vi "Read Data.vi"(8 "error in (no error)":errorcluster, 11 "DLP2 in":refnum<class "DLP2.lvclass">) -> (0 "error out":errorcluster, 2 "DLP2ReadData":T1, 3 "DLP2 out":refnum<class "DLP2.lvclass">)   [LabVIEW 2022 SP3, in "DLP2.lvclass"]
doc: "Developed by Kevin Thompson\nkevin@thompsonengineering.net\n\nCopyright 2018\nThompson Engineering, LLC"
uses:
  DLP2.lvclass
  DataTypes/Read Data--cluster.ctl
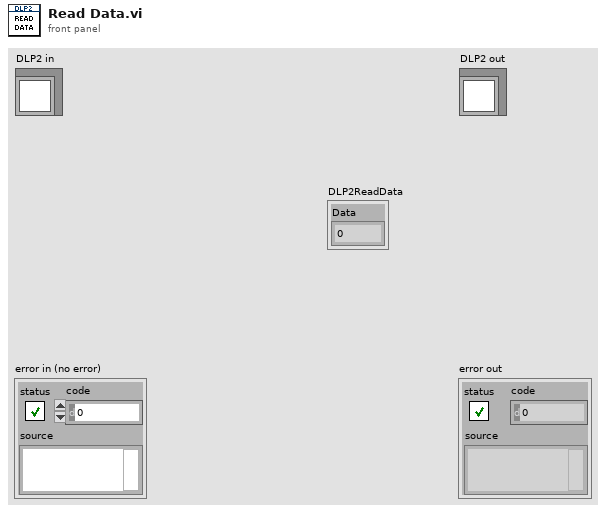
[diagram p1: front panel]
types:
  T1 = typedef "DLP2.lvclass/Read Data--cluster.ctl" = cluster{"Data":dbl}
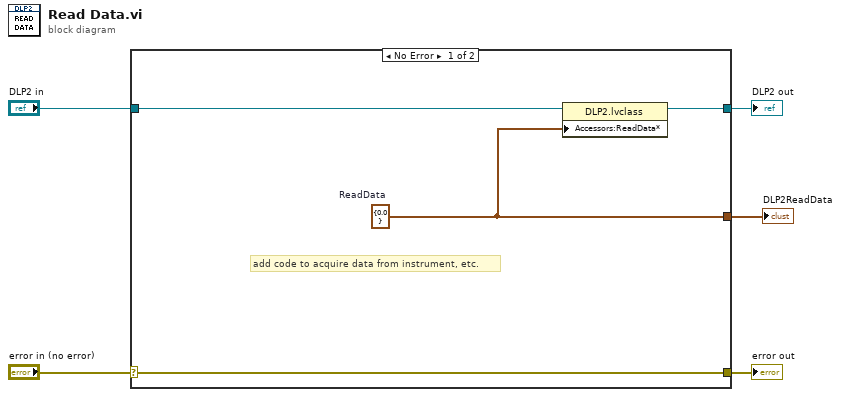
[diagram p0: block diagram]
diagram:
  n1 = case shown="No Error" "error in (no error)" {
    selector: "error in (no error)" -> [w9 w11]
    tunnel: [w9 w11] -> w4
    tunnel: [w7 w10] -> w2
    tunnel: "DLP2 in" -> [w8 w10]
    tunnel: [w6 _] -> w1
    frame No Error {
      w6 = T1 {"Data"=0.0}  # ReadData
      # "add code to acquire data from instrument, etc."
      n2 = property class="DLP2.lvclass"(reference=w8, "Accessors:ReadData*"=w6) -> (reference out=w7:refnum<class "DLP2.lvclass">)  [unwired: 1 in, 1 out]
    }
    frame Error {
    }
  }
  "error out" <- w4
  "DLP2 out" <- w2
  "DLP2ReadData" <- w1
